vi "TreeItemsCleared.vi"() -> (0 "error out":errorcluster)   [LabVIEW 2017, in "ResultTreeTest.lvlib" / "CreateResultTree.lvlib"]
uses:
  CreateResultTree.lvlib
  ResultTree/ResultTree.lvclass
  95cf8e39-8c85-4d1e-a934-2c249dc787aa.vi
panel:
  in  "Tree":string(tree)
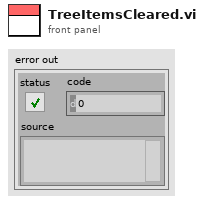
[diagram p1: front panel]
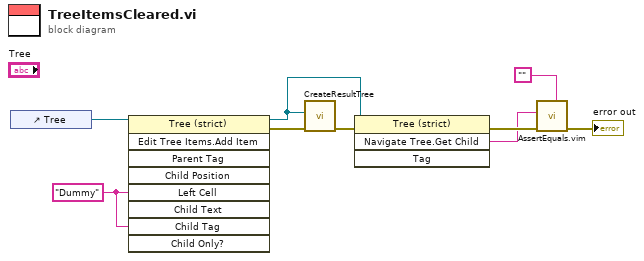
[diagram p0: block diagram]
diagram:
  w8 = "Dummy" ("Left Cell String")
  n1 = control-ref of="Tree"() -> (w9:refnum<vi>)
  n2 = invoke class="Tree (strict)" method="Edit Tree Items.Add Item"(reference=w9, "Left Cell"=w8, "Child Tag"=w8) -> (reference out=w5:refnum<vi>, error out=w7:errorcluster)  [unwired: 6 in, 7 out]
  n3 = call "CreateResultTree.vi"("error in (no error)"=w7, "Tree Refnum"=w5) -> ("error out"=w6:errorcluster)  [unwired: 8 in, 1 out]
  n4 = invoke class="Tree (strict)" method="Navigate Tree.Get Child"(reference=w5, error in=w6) -> (error out=w4:errorcluster, "Navigate Tree:Get Child"=w3:string)  [unwired: 2 in, 2 out]
  n5 = call "AssertEquals.vim"("Expected"="" ("Navigate Tree:Get Child"), "error in (no error)"=w4, "Actual"=w3) -> ("error out"=→"error out":errorcluster)  [unwired: 8 in]
